vi "GetParam.vi"(8 "error in (no error)":errorcluster caption="entrée d'erreur (pas d'erreur)", 11 "Spd_Matrix.lvclass":refnum<class "Spd_Matrix.lvclass">) -> (0 "error out":errorcluster caption="sortie d'erreur", 2 "make_spd_matrix":cluster{"n_dim":u32, "random_state":i32}={"n_dim"=1, "random_state"=-1} {"random_state" min=-1; "n_dim" min=1}, 3 "Spd_Matrix.lvclass":refnum<class "Spd_Matrix.lvclass">)   [LabVIEW 2020, in "Spd_Matrix.lvclass"]
doc: "Get Parameters"
uses:
  Spd_Matrix.lvclass
  Spd_Matrix.lvclass/Spd_Matrix.ctl
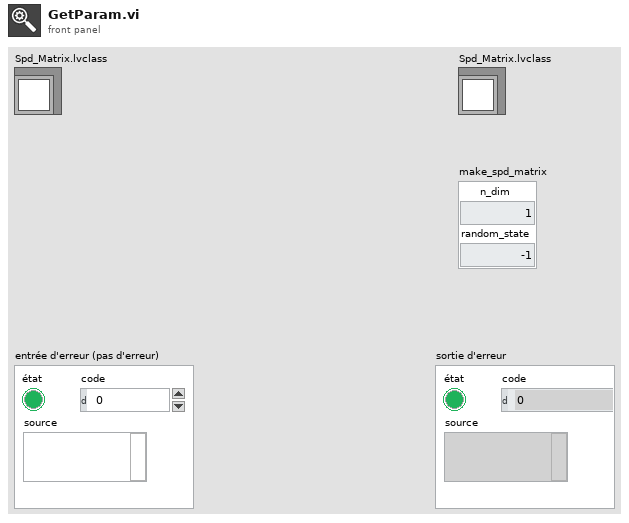
[diagram p1: front panel]
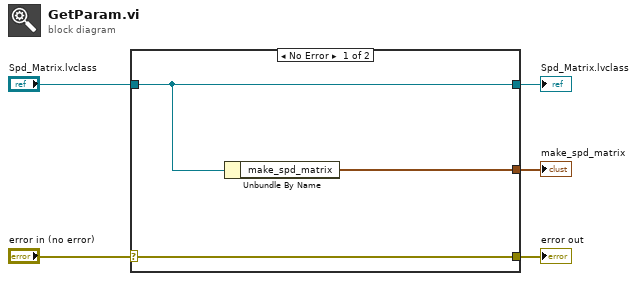
[diagram p0: block diagram]
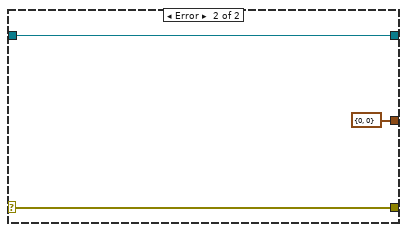
[diagram p2: hidden frame]
diagram:
  n1 = case shown="No Error" "error in (no error)" {
    selector: "error in (no error)" -> [w8 w10]
    tunnel: [w8 w10] -> w4
    tunnel: [w7 w11] -> w2
    tunnel: "Spd_Matrix.lvclass" -> [w7 w11]
    tunnel: [w6 cluster{"n_dim":u32, "random_state":i32} {"n_dim"=0, "random_state"=0} ("make_spd_matrix")] -> w1
    frame No Error {
      n2 = Unbundle By Name(w7) -> ("make_spd_matrix"=w6:cluster{"n_dim":u32, "random_state":i32})
    }
    frame Error {
    }
  }
  "error out" <- w4
  "Spd_Matrix.lvclass" <- w2
  "make_spd_matrix" <- w1
